vi "Workshop Exercise 3.vi"() -> ()   [LabVIEW 2019]
uses:
  <vilib>/ptbypt/NI_PtbyPt.lvlib
panel:
  out "Queue Loop Rate (ms)":dbl(knob) scale=0.0..100.0
  out "Local Variable Loop Rate (ms)":dbl(knob) scale=0.0..100.0
  out "Producer Loop Rate (ms)":dbl(knob) scale=0.0..100.0
  in  "Local Variable Loop Speed":u16(ring)=25 items=["Producer Loop Speed"=25, "Max. Speed"=0, "Twice as Producer"=12, "Half as Producer"=50, "1/10 as Producer"=250]
  in  "Queue Loop Speed":u16(ring)=25 items=["Producer Loop Speed"=25, "Max. Speed"=0, "Twice Producer Speed"=12, "Half Producer Speed"=50, "1/10 as Producer"=250]
  in  "Stop":bool
  out "Local Variable Loop":dbl(graph) caption="Local Variables Consumer Chart"
  out "Queue Loop":dbl(graph)=-9.510565162951542 caption="Queues Consumer Chart"
  out "Producer Loop":dbl(graph) caption="Producer Loop Chart"
  # "Producer Loop"
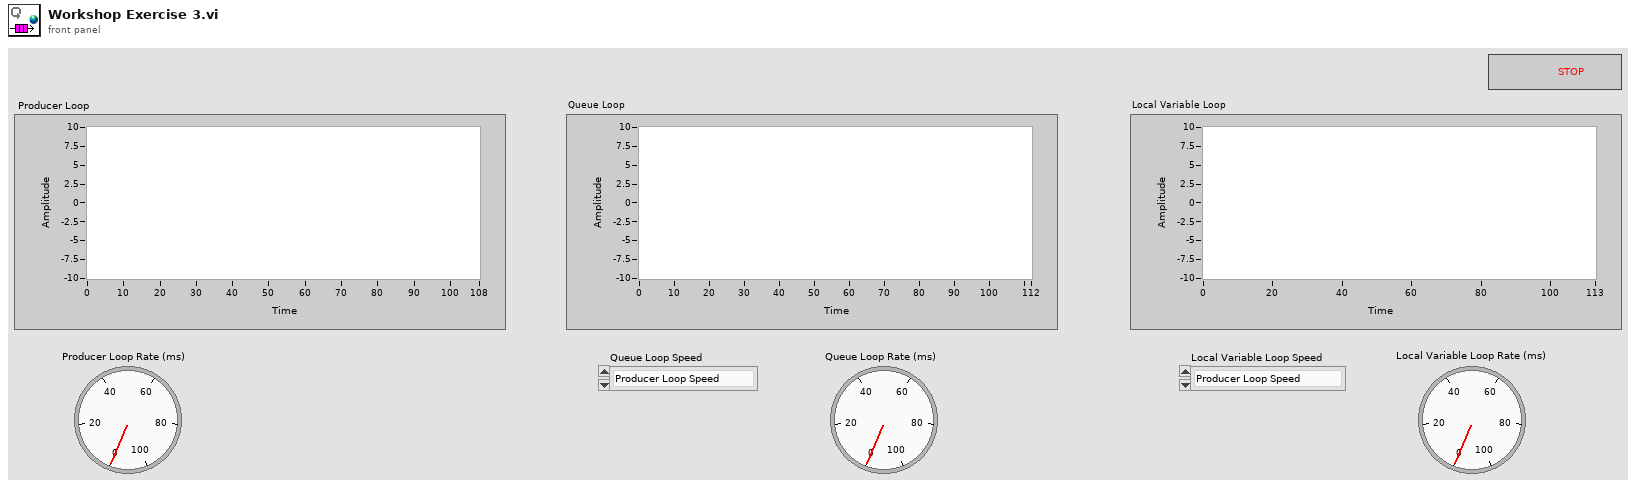
[diagram p1: front panel]
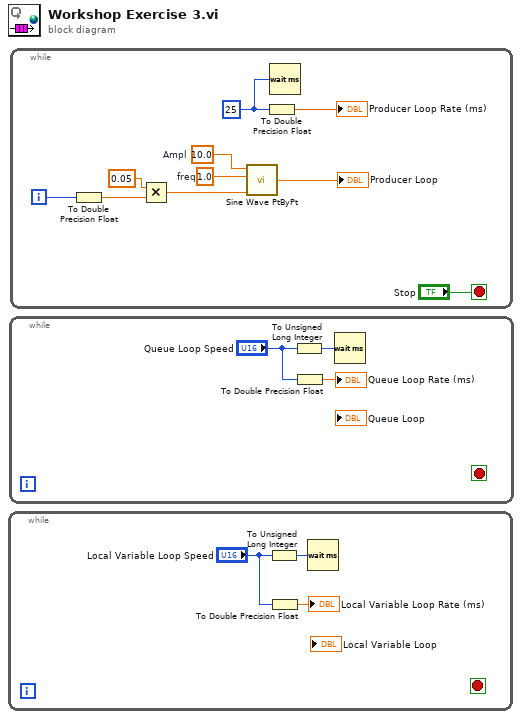
[diagram p0: block diagram]
diagram:
  n1 = while {
    stop <- _ stop-if-true
    # "Local Variable Consumer Loop"
    n2 = To Unsigned Long Integer(number="Local Variable Loop Speed") -> (unsigned 32bit integer=w3:u32)
    n3 = To Double Precision Float(number="Local Variable Loop Speed") -> (double precision float=→"Local Variable Loop Rate (ms)":dbl)
    n4 = Wait (ms)(milliseconds to wait=w3) -> ()  [unwired: 1 out]
  }
  n5 = while {
    stop <- _ stop-if-true
    # "Queue Consumer Loop"
    n6 = To Unsigned Long Integer(number="Queue Loop Speed") -> (unsigned 32bit integer=w6:u32)
    n7 = To Double Precision Float(number="Queue Loop Speed") -> (double precision float=→"Queue Loop Rate (ms)":dbl)
    n8 = Wait (ms)(milliseconds to wait=w6) -> ()  [unwired: 1 out]
  }
  n9 = while {
    i -> [w14]
    stop <- "Stop" stop-if-true
    w10 = 1.0  # freq
    w11 = 10.0  # Ampl
    w13 = u32 25 ("milliseconds to wait")
    # "Producer Loop"
    n10 = To Double Precision Float(number=w14) -> (double precision float=w7:dbl)
    n11 = Multiply(x=0.05 ("milliseconds to wait"), y=w7) -> (x*y=w8:dbl)
    n12 = call <vilib>:"Sine Wave PtByPt.vi"("time"=w8, "frequency"=w10, "amplitude"=w11) -> ("sine wave"=→"Producer Loop":dbl)  [unwired: 1 in]
    n13 = To Double Precision Float(number=w13) -> (double precision float=→"Producer Loop Rate (ms)":dbl)
    n14 = Wait (ms)(milliseconds to wait=w13) -> ()  [unwired: 1 out]
  }
